vi "Read Teller.vi"(11 "Msg in":refnum<class "Msg.lvclass">) -> (2 "Teller":refnum<class "Teller.lvclass">)   [LabVIEW 2025, in "jettl.lvlib" / "Msg.lvclass"]
uses:
  Msg.lvclass
  Teller/Teller.lvclass
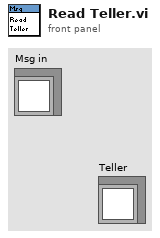
[diagram p1: front panel]
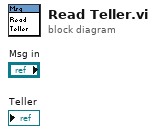
[diagram p0: block diagram]
diagram:
